vi "Test New Panel.vi"() -> ()   [LabVIEW 2012]
uses:
  Type Defs/Alt Display Large.ctl
  Type Defs/All Timers.ctl
  Type Defs/Timer Control.ctl
  Altitude/Altitude.xctl
  Type Defs/Action Time.ctl
  Mode Control/Mode.xctl
  Type Defs/Alt Control.ctl
  Type Defs/Alt Digit 100 New.ctl
panel:
  out "Mode  3":enum16{"Run", "Hold", "Off"}(ring)=enum."Off"
  in  "Main States":T1(tab)=enum."Detailed Display"
  out "ALT DISPLAY":T2 format="%#_5f"
  out "Altitude Message":string
  in  "Confirm Now 2":bool
  in  "ALT SET 2":T3 {"Alt Digit 100" min=0 max=9 step=1; "Alt Digit 100" min=0 max=9 step=1; "Alt Digit 100" min=0 max=9 step=1; "Alt Digit 100" min=0 max=9 step=1; "Alt Digit 100" min=0 max=9 step=1}
  in  "Mode 2":cluster{"Run":bool, "Hold":bool, "Off":bool}={"Run"=FALSE, "Hold"=TRUE, "Off"=FALSE}
  out "ALT DISPLAY 2":T2 format="%#_5f"
  in  "Add Note":bool
  in  "Confirm Now":bool
  in  "Notes":string
  in  "ALT SET":T3 {"Alt Digit 100" min=0 max=9 step=1; "Alt Digit 100" min=0 max=9 step=1; "Alt Digit 100" min=0 max=9 step=1; "Alt Digit 100" min=0 max=9 step=1; "Alt Digit 100" min=0 max=9 step=1}
  out "Altitude":sgl
  in  "Mode":cluster{"Run":bool, "Hold":bool, "Off":bool}={"Run"=FALSE, "Hold"=TRUE, "Off"=FALSE}
  in  "Timers":T5 {"Timer 4"."Action Time" format="%<%H:%M>t"; "Timer 3"."Action Time" format="%<%H:%M>t"; "Timer 2"."Action Time" format="%<%H:%M>t"; "Timer"."Action Time" format="%<%H:%M>t"}
  in  "Datalog File":path
  # "Current Effective Altitude in  Meters"
  # "BETA  0.01"
  # "M\nE\nT\nE\nR\nS"
  # "%"
  # "1"
  # "1"
  # "1"
  # "1"
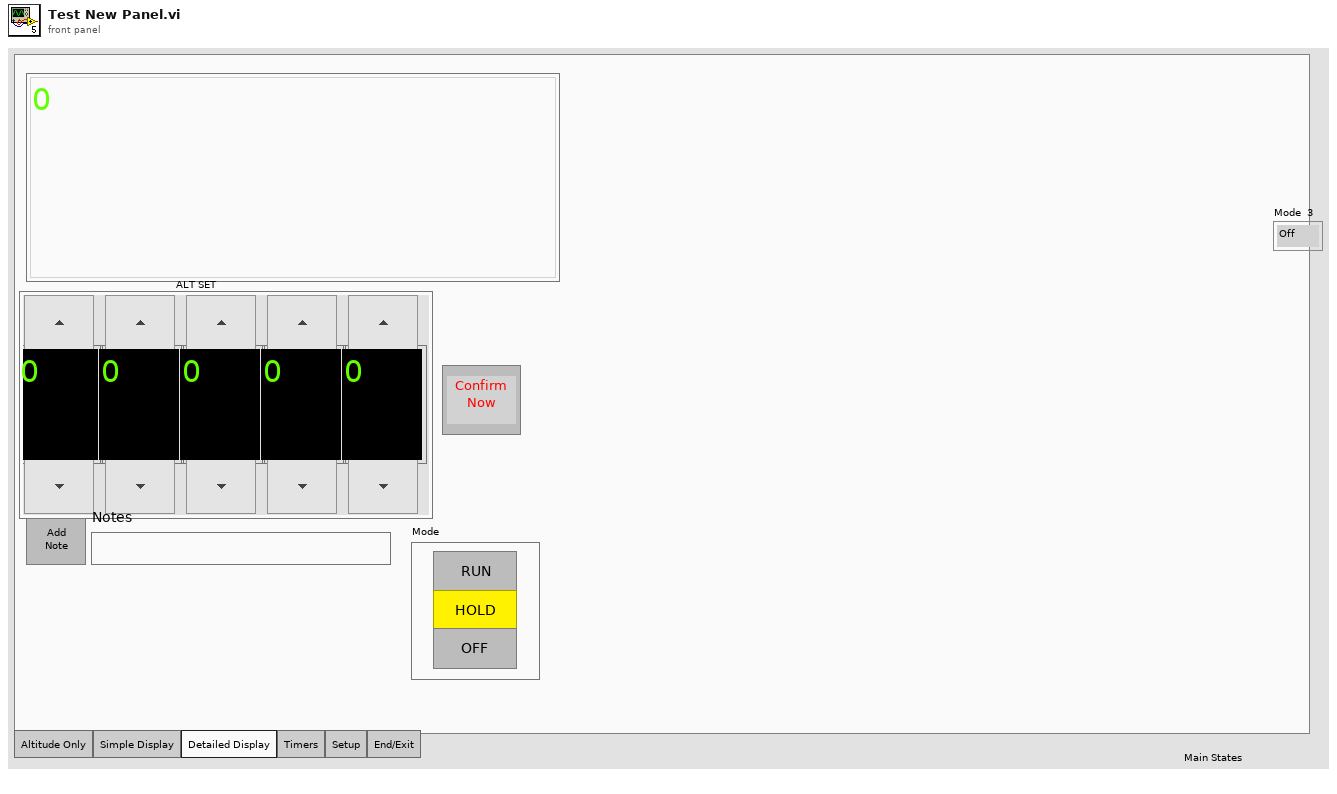
[diagram p1: front panel]
types:
  T1 = enum32{"Altitude Only", "Simple Display", "Detailed Display", "Timers", "Setup", "End/Exit"}
  T2 = typedef "Alt Display Large.ctl" = sgl
  T3 = typedef "Alt Control.ctl" = cluster{"Alt Digit 100":T4, "Alt Digit 100":T4, "Alt Digit 100":T4, "Alt Digit 100":T4, "Alt Digit 100":T4}
  T4 = typedef "Alt Digit 100 New.ctl" = i8
  T5 = typedef "All Timers.ctl" = cluster{"Timer":T6, "Timer 2":T6, "Timer 3":T6, "Timer 4":T6}
  T6 = typedef "Timer Control.ctl" = cluster{"Sun":bool, "Timer":bool, "Altitude":sgl, "Action Time":T7, "Mon":bool, "Tues":bool, "Wed":bool, "Thur":bool, "Fri":bool, "Sat":bool, "Mode":enum8{"Off", "Stby", "Hold", "Run"}}
  T7 = typedef "Action Time.ctl" = dbl
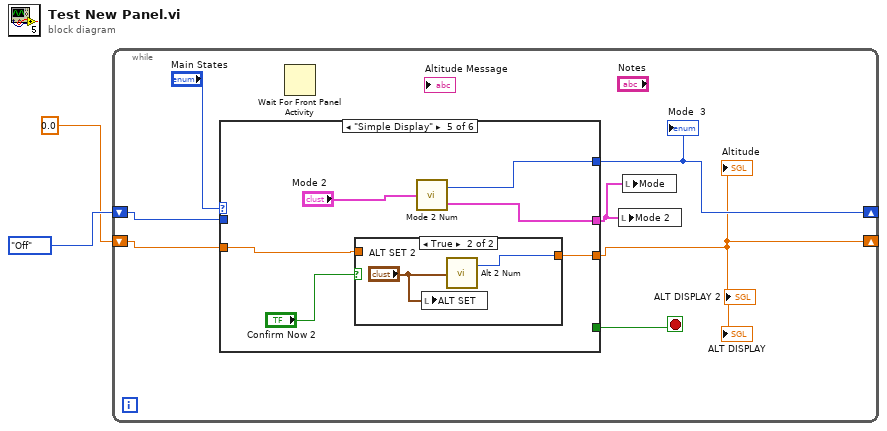
[diagram p0: block diagram]
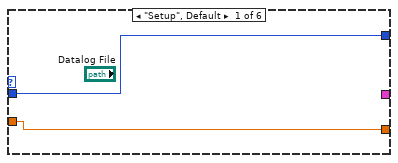
[diagram p2: hidden frame]
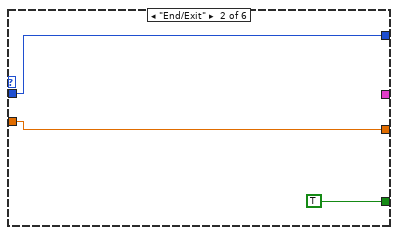
[diagram p3: hidden frame]
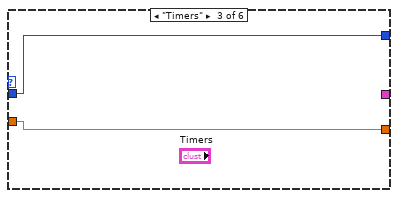
[diagram p4: hidden frame]
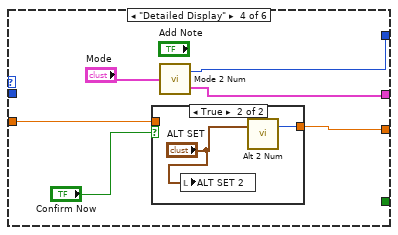
[diagram p5: hidden frame]
diagram:
  n1 = while {
    shift-right: [w7] -> _
    shift-left: enum16{"Run", "Hold", "Off"}."Off" ("Mode") -> [w6]
    shift-right: [w4] -> _
    shift-left: sgl 0.0 ("Alt") -> [w5]
    stop <- w8 stop-if-true
    n2 = case shown="\"Simple Display\"" "Main States" {
      tunnel: [_ TRUE ("stop") _ _ _ _] -> w8
      tunnel: [w10 w12 w15 w21 w30 w35] -> w4
      tunnel: [w11 w13 w16 w20 w29 w36] -> w7
      tunnel: w6 -> [w11 w13 w16 _ _ w36]
      tunnel: w5 -> [w10 w12 w15 w18 w27 w35]
      tunnel: [_ _ _ w17 w26 _] -> w3
      frame "Setup", Default {
      }
      frame "End/Exit" {
      }
      frame "Timers" {
      }
      frame "Detailed Display" {
        n3 = case shown="True" "Confirm Now" {
          tunnel: [w23 w25] -> w21
          tunnel: w18 -> [w23 _]
          frame False {
          }
          frame True {
            n4 = local write "ALT SET 2"("ALT SET") -> ()
            n5 = call "Alt 2 Num.vi"("Alt Ctl"="ALT SET") -> ("Alt"=w25:i32)  [unwired: 2 in]
          }
        }
        n6 = call "Mode 2 Num.vi"("Mode"="Mode") -> ("Mode"=w20:enum16{"Run", "Hold", "Off"}, "Mode Out"=w17:cluster{"Run":bool, "Hold":bool, "Off":bool})
      }
      frame "Simple Display" {
        n7 = case shown="True" "Confirm Now 2" {
          tunnel: [w32 w34] -> w30
          tunnel: w27 -> [w32 _]
          frame False {
          }
          frame True {
            n8 = local write "ALT SET"("ALT SET 2") -> ()
            n9 = call "Alt 2 Num.vi"("Alt Ctl"="ALT SET 2") -> ("Alt"=w34:i32)  [unwired: 2 in]
          }
        }
        n10 = call "Mode 2 Num.vi"("Mode"="Mode 2") -> ("Mode"=w29:enum16{"Run", "Hold", "Off"}, "Mode Out"=w26:cluster{"Run":bool, "Hold":bool, "Off":bool})
      }
      frame "Altitude Only" {
      }
    }
    "Mode  3" <- w7
    "ALT DISPLAY" <- w4
    "ALT DISPLAY 2" <- w4
    "Altitude" <- w4
    n11 = Wait For Front Panel Activity() -> ()  [unwired: 3 in, 1 out]
    n12 = local write "Mode 2"(w3) -> ()
    n13 = local write "Mode"(w3) -> ()
  }
